vi "DFF.vi"(2 "Clock":bool, 3 "D":bool) -> (0 "Q Roof":bool, 1 "Q":bool)   [LabVIEW 2012]
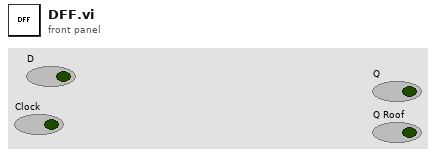
[diagram p1: front panel]
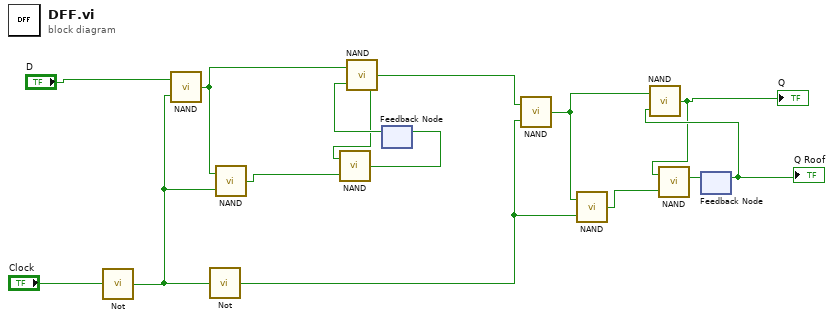
[diagram p0: block diagram]
diagram:
  n1 = call "Not.vi"("In"="Clock") -> ("Out"=w12:bool)
  n2 = call "NAND.vi"("b"=w12, "a"="D") -> ("x"=w11:bool)
  n3 = call "Not.vi"("In"=w12) -> ("Out"=w6:bool)
  n4 = call "NAND.vi"("b"=w12, "a"=w11) -> ("x"=w10:bool)
  n5 = feedback #1() -> (w8:bool)  [unwired: 1 in]
  n6 = call "NAND.vi"("b"=w8, "a"=w11) -> ("x"=w7:bool)
  n7 = call "NAND.vi"("b"=w10, "a"=w7) -> ("x"=w9:bool)
  n8 = feedback-in #1(w9) -> ()
  n9 = call "NAND.vi"("b"=w6, "a"=w7) -> ("x"=w5:bool)
  n10 = call "NAND.vi"("b"=w6, "a"=w5) -> ("x"=w4:bool)
  n11 = feedback #2() -> (w2:bool)  [unwired: 1 in]
  "Q Roof" <- w2
  n12 = call "NAND.vi"("b"=w2, "a"=w5) -> ("x"=w1:bool)
  "Q" <- w1
  n13 = call "NAND.vi"("b"=w4, "a"=w1) -> ("x"=w3:bool)
  n14 = feedback-in #2(w3) -> ()
